vi "Get All VIs Measured.vi"(8 "error in (no error)":errorcluster, 11 "CodeCoverage in":refnum<class "Code Coverage.lvclass">) -> (0 "error out":errorcluster, 2 "All VIs Measured":path[](array[path]), 3 "CodeCoverage out":refnum<class "Code Coverage.lvclass">)   [LabVIEW 2017, in "Code Coverage.lvclass"]
doc: "Returns the paths of all VIs for which code coverage data is available."
uses:
  Code Coverage.lvclass
  Code Coverage.lvclass/Code Coverage.ctl
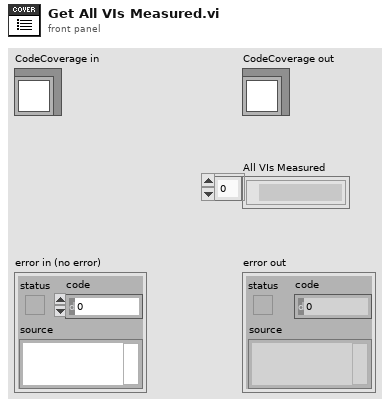
[diagram p1: front panel]
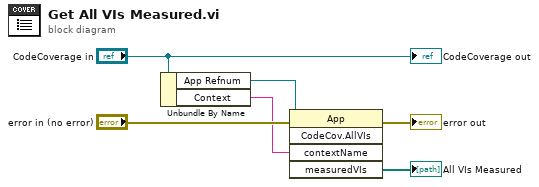
[diagram p0: block diagram]
diagram:
  n1 = Unbundle By Name("CodeCoverage in") -> ("App Refnum"=w3:refnum<vi>, "Context"=w2:string)
  n2 = invoke class="App" method="CodeCov.AllVIs"(reference=w3, error in="error in (no error)", "contextName"=w2) -> (error out=→"error out":errorcluster, "measuredVIs"=→"All VIs Measured":path[])  [unwired: 2 in, 3 out]
  "CodeCoverage out" <- "CodeCoverage in"
